vi "drivePID.vi"() -> ()   [LabVIEW 2012]
uses:
  <vilib>/Rock Robotics/WPI/Joystick/WPI_JoystickAxis.ctl
  <vilib>/Rock Robotics/WPI/Joystick/WPI_JoystickGetSetRefNum.vi
  Robot Global Data.vi
  <vilib>/addons/control/pid/pid.llb/PID (DBL).vi
  <vilib>/addons/control/pid/NI_PID_pid.lvlib
panel:
  in  "output range RIGHT":cluster{"output high":dbl, "output low":dbl}={"output high"=100.0, "output low"=-100.0} {"output low" format="%.2f"; "output high" format="%.2f"}
  in  "output range LEFT":cluster{"output high":dbl, "output low":dbl}={"output high"=100.0, "output low"=-100.0} {"output low" format="%.2f"; "output high" format="%.2f"}
  in  "PID RIGHT":T1={"proportional gain (Kc)"=1.0, "integral time (Ti, min)"=0.01, "derivative time (Td, min)"=0.0} {"derivative time (Td, min)" format="%.3f"; "integral time (Ti, min)" format="%.3f"; "proportional gain (Kc)" format="%.3f"}
  in  "PID LEFT":T1={"proportional gain (Kc)"=1.0, "integral time (Ti, min)"=0.01, "derivative time (Td, min)"=0.0} {"derivative time (Td, min)" format="%.3f"; "integral time (Ti, min)" format="%.3f"; "proportional gain (Kc)" format="%.3f"}
  in  "stop":bool
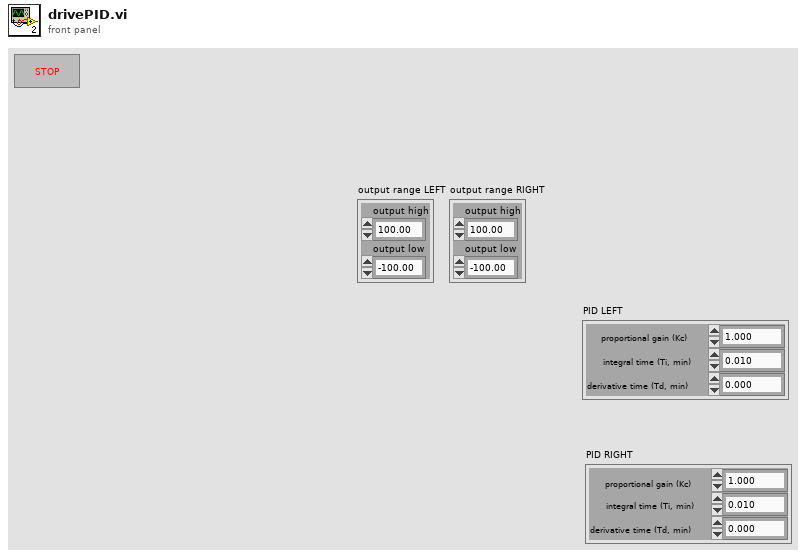
[diagram p1: front panel]
types:
  T1 = cluster{"proportional gain (Kc)":dbl, "integral time (Ti, min)":dbl, "derivative time (Td, min)":dbl}
  T2 = typedef "WPI_JoystickDevRef.ctl" = cluster{"Device":T3}
  T3 = typedef "WPI_JoystickDeviceEnum.ctl" = enum16{"USB 1", "USB 2", "USB 3", "USB 4", "Kinect 1", "Kinect 2"}
  T4 = typedef "WPI_EncoderDevRef.ctl" = cluster{"DevStatus":errorcluster, "EncoderIndex":T5, "CounterIndex":T6, "DistancePerCount":dbl, "Decoding Type":T7}
  T5 = typedef "FPGA_EncoderIdx.ctl" = enum8{"Enc 0", "Enc 1", "Enc 2", "Enc 3", "Invalid"}
  T6 = typedef "FPGA_CounterCtrSystemIndex.ctl" = enum8{"Ctr 0", "Ctr 1", "Ctr 2", "Ctr 3", "Ctr 4", "Ctr 5", "Ctr 6", "Ctr 7", "Invalid"}
  T7 = typedef "WPI_EncoderType.ctl" = enum16{"1x", "2x", "4x"}
  T8 = typedef "WPI_JoystickAxis.ctl" = enum16{"Axis 1", "Axis 2", "Axis 3", "Axis 4", "Axis 5", "Axis 6"}
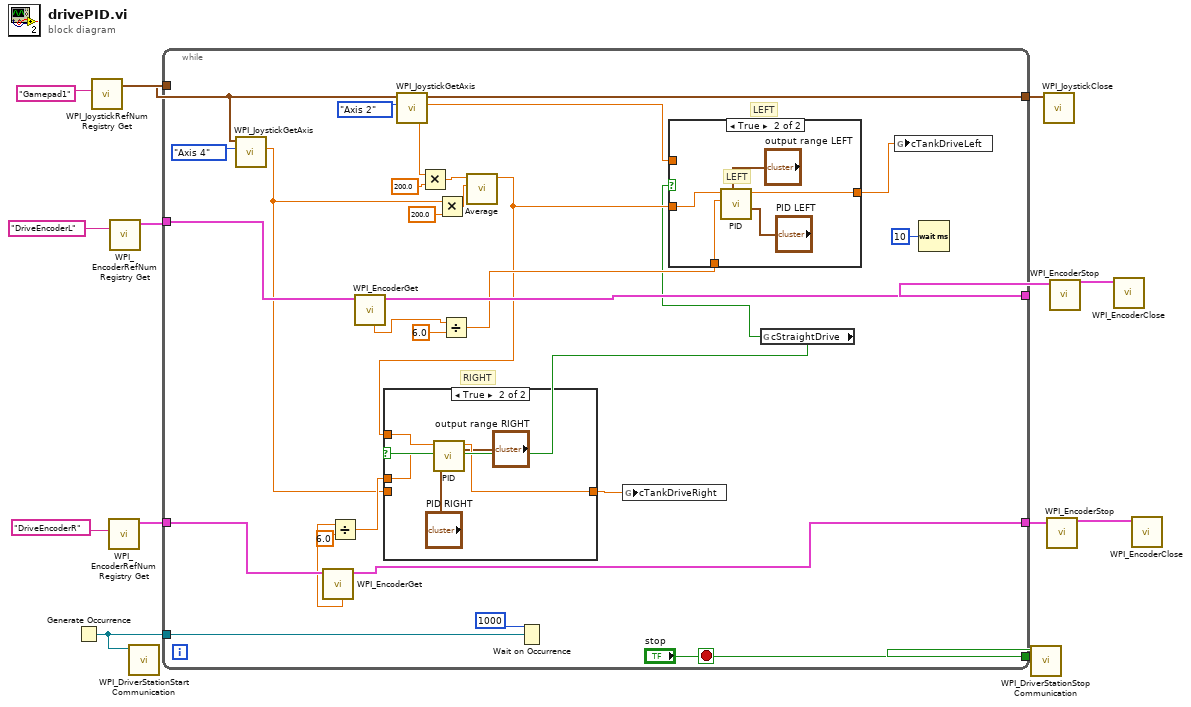
[diagram p0: block diagram]
diagram:
  n1 = Generate Occurrence() -> (w13:refnum<k4>)
  n2 = call <vilib>:"WPI_JoystickRefNum Registry Get.vi"("refnum name"="Gamepad1") -> ("JoystickDevRef"=w1:T2)  [unwired: 9 in, 1 out]
  n3 = call <vilib>:"WPI_EncoderRefNum Registry Get.vi"("refnum name"="DriveEncoderR") -> ("EncoderDevRef"=w3:T4)  [unwired: 9 in, 1 out]
  n4 = call <vilib>:"WPI_EncoderRefNum Registry Get.vi"("refnum name"="DriveEncoderL") -> ("EncoderDevRef"=w5:T4)  [unwired: 9 in, 1 out]
  n5 = call <vilib>:"WPI_DriverStationStart Communication.vi"("occurrence"=w13) -> ()  [unwired: 11 out]
  n6 = while {
    tunnel: w13 -> [w41]
    tunnel: ["stop"] -> w12
    tunnel: w1 -> [w35]
    tunnel: [w19] -> w11
    tunnel: w5 -> [w37]
    tunnel: [w36] -> w8
    tunnel: w3 -> [w33]
    tunnel: [w32] -> w10
    stop <- "stop" stop-if-true
    # "RIGHT"
    # "LEFT"
    n7 = call <vilib>:"WPI_JoystickGetAxis.vi"("Axis"=WPI_JoystickAxis."Axis 4", "JoystickDevRef"=w35) -> ("Value"=w18:dbl)  [unwired: 8 in, 1 out]
    n8 = call <vilib>:"WPI_EncoderGet.vi"("EncoderDevRef"=w33) -> ("EncoderDevRef"=w32:T4, "Rate"=w23:dbl)  [unwired: 5 in, 4 out]
    n9 = Divide(x=w23, y=6.0) -> (x/y=w21:dbl)
    n10 = call <vilib>:"WPI_EncoderGet.vi"("EncoderDevRef"=w37) -> ("EncoderDevRef"=w36:T4, "Rate"=w31:dbl)  [unwired: 5 in, 4 out]
    n11 = call <vilib>:"WPI_JoystickGetAxis.vi"("Axis"=WPI_JoystickAxis."Axis 2", "JoystickDevRef"=w35) -> ("Value"=w25:dbl, "JoystickDevRef"=w19:T2)  [unwired: 8 in]
    n12 = Multiply(x=w25, y=200.0) -> (x*y=w26:dbl)
    n13 = Multiply(x=w18, y=200.0) -> (x*y=w20:dbl)
    n14 = Divide(x=w31, y=6.0) -> (x/y=w29:dbl)
    n15 = call "Average.vi"("y"=w20, "x"=w26) -> ("x/y"=w22:dbl)  [unwired: 9 in]
    n16 = Wait on Occurrence(2:w41, 3:1000 ("ms timeout (-1)")) -> ()  [unwired: 2 out]
    n17 = global read "Robot Global Data.vi" "cStraightDrive"() -> (w17:bool)
    n18 = case shown="True" w17 {
      tunnel: w22 -> [_ w47]
      tunnel: w21 -> [_ w46]
      tunnel: [w42 w45] -> w15
      tunnel: w18 -> [w42 _]
      frame False {
      }
      frame True {
        n19 = call-poly <vilib>:"PID.vi"("output range"="output range RIGHT", "PID gains"="PID RIGHT", "process variable"=w46, "setpoint"=w47) -> ("output"=w45:dbl)  [unwired: 6 in, 1 out]
      }
    }
    n20 = global write "Robot Global Data.vi" "cTankDriveRight"(w15) -> ()
    n21 = case shown="True" w17 {
      tunnel: w22 -> [_ w53]
      tunnel: w29 -> [_ w52]
      tunnel: [w48 w51] -> w14
      tunnel: w25 -> [w48 _]
      frame False {
      }
      frame True {
        # "LEFT"
        n22 = call-poly <vilib>:"PID.vi"("output range"="output range LEFT", "PID gains"="PID LEFT", "process variable"=w52, "setpoint"=w53) -> ("output"=w51:dbl)  [unwired: 6 in, 1 out]
      }
    }
    n23 = global write "Robot Global Data.vi" "cTankDriveLeft"(w14) -> ()
    n24 = Wait (ms)(milliseconds to wait=u32 10) -> ()  [unwired: 1 out]
  }
  n25 = call <vilib>:"WPI_DriverStationStop Communication.vi"("StopCommunication"=w12) -> ()  [unwired: 1 in, 10 out]
  n26 = call <vilib>:"WPI_JoystickClose.vi"("JoystickDevRef"=w11) -> ()  [unwired: 11 in]
  n27 = call <vilib>:"WPI_EncoderStop.vi"("EncoderDevRef"=w10) -> ("EncoderDevRef"=w9:T4)  [unwired: 9 in, 1 out]
  n28 = call <vilib>:"WPI_EncoderStop.vi"("EncoderDevRef"=w8) -> ("EncoderDevRef"=w7:T4)  [unwired: 9 in, 1 out]
  n29 = call <vilib>:"WPI_EncoderClose.vi"("EncoderDevRef"=w7) -> ()  [unwired: 10 in, 1 out]
  n30 = call <vilib>:"WPI_EncoderClose.vi"("EncoderDevRef"=w9) -> ()  [unwired: 10 in, 1 out]
